vi "Bandpass filter edit.vi"(6 "Fr":dbl, 8 "C":dbl, 9 "L":dbl, 10 "R":dbl, 11 "Circuit Type":T1) -> (1 "Fl":dbl, 2 "Fh":dbl, 3 "half":dbl)   [LabVIEW 2017]
uses:
  Types/Circuit Type Enum.ctl
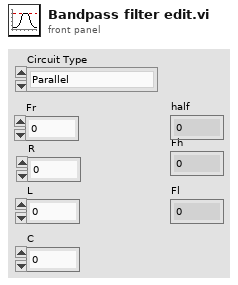
[diagram p1: front panel]
types:
  T1 = typedef "Circuit Type Enum.ctl" = enum16{"Parallel", "Serial"}
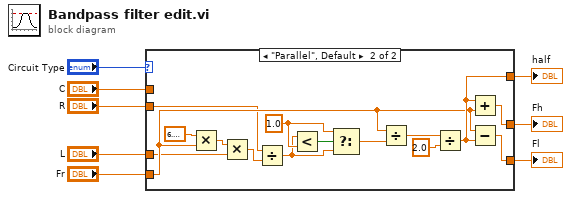
[diagram p0: block diagram]
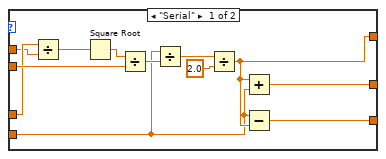
[diagram p2: hidden frame]
diagram:
  n1 = case shown="\"Parallel\", Default" "Circuit Type" {
    tunnel: [w13 w32] -> w8
    tunnel: [w15 w25] -> w7
    tunnel: [w14 w24] -> w6
    tunnel: "Fr" -> [w12 w23]
    tunnel: "L" -> [w10 w22]
    tunnel: "R" -> [w11 w21]
    tunnel: "C" -> [w9 _]
    frame "Serial" {
      n2 = Divide(x=w10, y=w9) -> (x/y=w17:dbl)
      n3 = Square Root(x=w17) -> (sqrt(x)=w16:dbl)
      n4 = Divide(x=w16, y=w11) -> (x/y=w20:dbl)
      n5 = Divide(x=w12, y=w20) -> (x/y=w19:dbl)
      n6 = Divide(x=w19, y=2.0) -> (x/y=w13:dbl)
      n7 = Add(x=w13, y=w12) -> (x+y=w15:dbl)
      n8 = Subtract(x=w12, y=w13) -> (x-y=w14:dbl)
    }
    frame "Parallel", Default {
      w29 = 1.0 ("y")
      n9 = Multiply(x=6.283185307179586, y=w23) -> (x*y=w34:dbl)
      n10 = Multiply(x=w34, y=w22) -> (x*y=w31:dbl)
      n11 = Divide(x=w21, y=w31) -> (x/y=w28:dbl)
      n12 = Less?(x=w28, y=w29) -> (x < y?=w30:bool)
      n13 = Select(t=w29, s=w30, f=w28) -> (s? t:f=w27:dbl)
      n14 = Divide(x=w23, y=w27) -> (x/y=w26:dbl)
      n15 = Divide(x=w26, y=2.0) -> (x/y=w32:dbl)
      n16 = Add(x=w32, y=w23) -> (x+y=w25:dbl)
      n17 = Subtract(x=w23, y=w32) -> (x-y=w24:dbl)
    }
  }
  "Fh" <- w7
  "Fl" <- w6
  "half" <- w8
